vi "mm to in conversion.vi"(1 "mm":i16) -> (0 "in":i16)   [LabVIEW 2010]
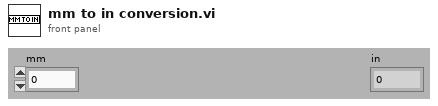
[diagram p1: front panel]
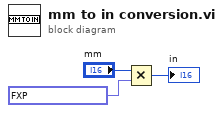
[diagram p0: block diagram]
diagram:
  n1 = Multiply(x="mm", y=fxp<+,16,1> 0.03936767578125) -> (x*y=→"in":i16)
